vi "Get Source Configuration List Catalog.vi"(8 "error in (no error)":errorcluster, 11 "VISA resource name":refnum<visa-resource-name>) -> (0 "error out":errorcluster, 2 "Source Configuration List Catalog":string, 3 "VISA resource name out":refnum<visa-resource-name>)   [LabVIEW 2021, in "Keithley 2450.lvlib"]
doc: "This gets the Source configuration list catalog.\n\nThis gets one name each time. This returns NULL to indicate that there are no more names to return. If this returns NULL the first time then no measure configuration lists have been created for the instrument."
uses:
  Keithley 2450.lvlib
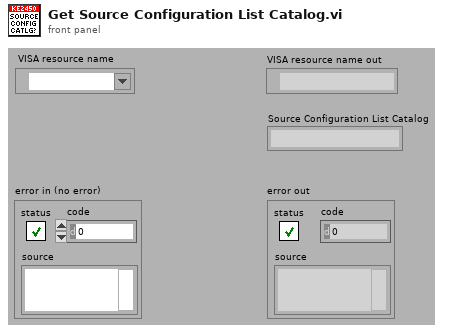
[diagram p1: front panel]
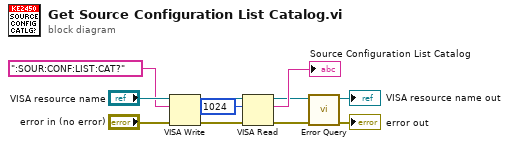
[diagram p0: block diagram]
diagram:
  n1 = VISA Write(VISA resource name="VISA resource name", write buffer=":SOUR:CONF:LIST:CAT?", error in (no error)="error in (no error)") -> (VISA resource name out=w10:refnum<visa-resource-name>, error out=w11:errorcluster)  [unwired: 1 out]
  n2 = VISA Read(VISA resource name=w10, byte count=u32 1024, error in (no error)=w11) -> (VISA resource name out=w2:refnum<visa-resource-name>, read buffer=→"Source Configuration List Catalog":string, error out=w1:errorcluster)  [unwired: 1 out]
  n3 = call "Error Query.vi"("error in (no error)"=w1, "VISA resource name"=w2) -> ("error out"=→"error out":errorcluster, "VISA resource name out"=→"VISA resource name out":refnum<visa-resource-name>)  [unwired: 8 out]
